vi "Results.vi"(8 "error in (no error)":errorcluster, 11 "PmuDelayClass in":refnum<class "PmuDelay.lvclass">) -> (0 "error out":errorcluster, 3 "PmuDelayClass out":refnum<class "PmuDelay.lvclass">)   [LabVIEW 2018, in "AnalysisPlugins.lvlib" / "PmuDelay.lvclass"]
uses:
  PmuDelay.lvclass
  C:/projects/ICDAS/NistPluggableModules/Analysis/AnalysisPlugins/AnalysisPluginBaseClass/AnalysisPluginsBase.lvclass
  C:/projects/ICDAS/NistPluggableModules/Analysis/AnalysisPlugins/PmuAnalysisClass/PmuAnalysis.lvclass
  AnalysisPluginBaseClass/AnalysisPluginsBase.lvclass/AnalysisPluginsBase.ctl
  PmuAnalysisClass/PmuAnalysis.lvclass/PmuAnalysis.ctl
  PmuAnalysisClass/Accessors/Read PmuReport.vi
  PmuAnalysisClass/Accessors/Read Reference.vi
  AnalysisPluginBaseClass/Accessors/Write Result.vi
  AnalysisPluginBaseClass/Accessors/Read Window.vi
  AnalysisPluginBaseClass/AnalysisPluginsBase.lvclass
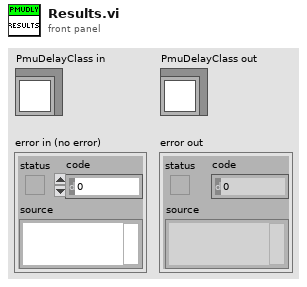
[diagram p1: front panel]
types:
  T1 = typedef "AnalysisPlugins.lvlib/AnalysisPluginsBase.lvclass/clWindowData.ctl" = cluster{"Timestamp":ext, "Samples":dbl[][], "Window Valid":bool, "T0":ext}
  T2 = typedef "AnalysisPlugins.lvlib/PmuAnalysis.lvclass/PmuData.ctl" = cluster{"Timestamp":dbl, "Synx":cdb[], "Freq":dbl, "ROCOF":dbl, "ID":i16}
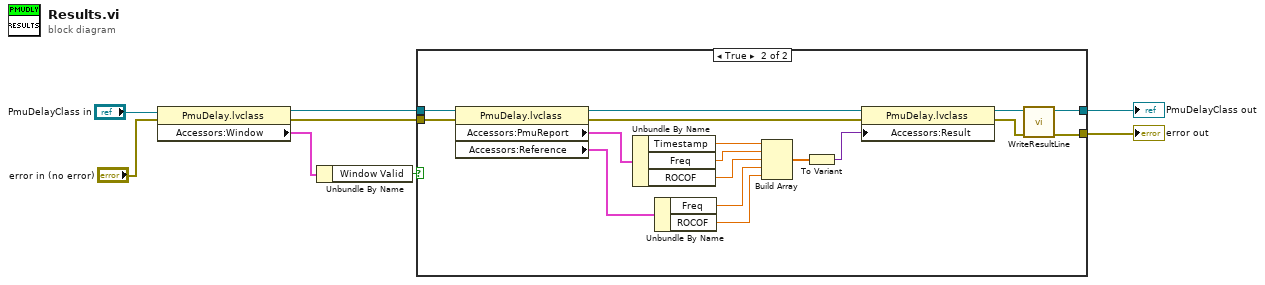
[diagram p0: block diagram]
diagram:
  n1 = property class="PmuDelay.lvclass"(reference="PmuDelayClass in", error in="error in (no error)") -> (reference out=w4:refnum<class "PmuDelay.lvclass">, error out=w3:errorcluster, "Accessors:Window"=w6:T1)
  n2 = Unbundle By Name(w6) -> ("Window Valid"=w5:bool)
  n3 = case shown="True" w5 {
    tunnel: w4 -> [w10 w27]
    tunnel: w3 -> [w9 w19]
    tunnel: [w10 w13] -> w2
    tunnel: [w9 w11] -> w1
    frame False {
    }
    frame True {
      n4 = property class="PmuDelay.lvclass"(reference=w27, error in=w19) -> (reference out=w17:refnum<class "PmuDelay.lvclass">, error out=w16:errorcluster, "Accessors:PmuReport"=w26:T2, "Accessors:Reference"=w25:T2)
      n5 = Unbundle By Name(w26) -> ("Timestamp"=w24:dbl, "Freq"=w23:dbl, "ROCOF"=w22:dbl)
      n6 = Unbundle By Name(w25) -> ("Freq"=w21:dbl, "ROCOF"=w20:dbl)
      n7 = Build Array(w24, w23, w22, w21, w20) -> (w18:dbl[])
      n8 = To Variant(anything=w18) -> (Variant=w15:variant)
      n9 = property class="PmuDelay.lvclass"(reference=w17, error in=w16, "Accessors:Result"=w15) -> (reference out=w14:refnum<class "PmuDelay.lvclass">, error out=w12:errorcluster)
      n10 = call "WriteResultLine.vi"("error in (no error)"=w12, "AnalysisPluginsBase in"=w14) -> ("error out"=w11:errorcluster, "AnalysisPluginsBase out"=w13:refnum<class "PmuDelay.lvclass">)  [unwired: 8 in]
    }
  }
  "error out" <- w1
  "PmuDelayClass out" <- w2
